vi "题目七.vi"() -> ()   [LabVIEW 2017]
uses:
  <vilib>/Utility/file.llb/Read Delimited Spreadsheet (DBL).vi
  <vilib>/Analysis/NI_AALBase.lvlib
panel:
  out "波形图表":dbl(graph)
  out "all rows":dbl[][](array[numeric]) caption="所有行"
  in  "cycles":dbl=1.0 caption="周期" format="%0.2f"
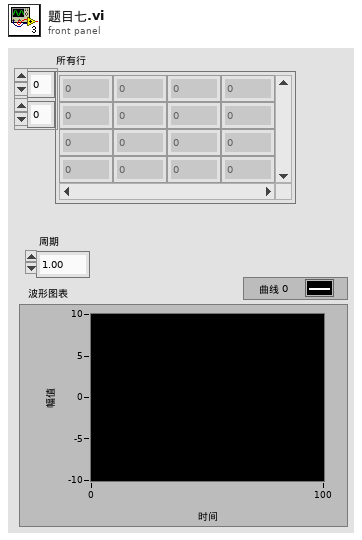
[diagram p1: front panel]
types:
  T1 = enum16{"open", "replace", "create", "open or create", "replace or create", "replace or create with confirmation"}
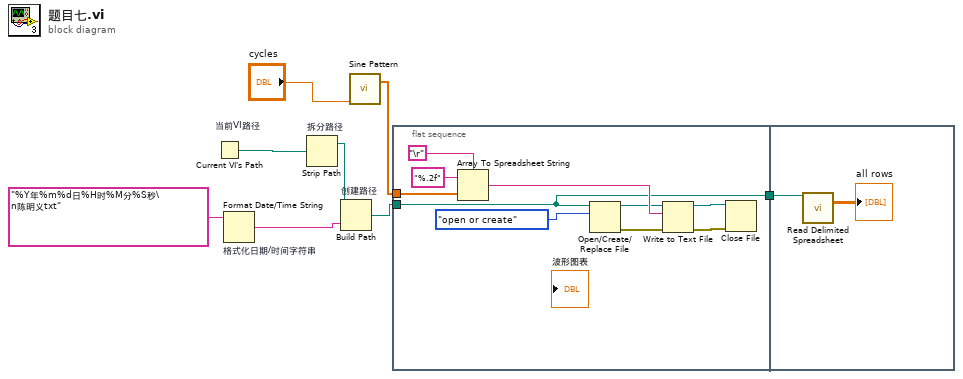
[diagram p0: block diagram]
diagram:
  n1 = Current VI's Path "当前VI路径"() -> (path=w8:path)
  n2 = Format Date/Time String "格式化日期/时间字符串"(time format string (%c)="%Y年%m%d日%H时%M分%S秒\n陈明义txt") -> (date/time string=w7:string)  [unwired: 2 in]
  n3 = Strip Path "拆分路径"(path=w8) -> (stripped path=w6:path)  [unwired: 1 out]
  n4 = Build Path "创建路径"(base path=w6, name or relative path=w7) -> (appended path=w3:path)
  n5 = call <vilib>:"Sine Pattern.vi"("cycles"="cycles") -> ("Sinusoidal Pattern"=w2:dbl[])  [unwired: 3 in, 1 out]
  n6 = flat-sequence {
    tunnel: w3 -> [w10]
    tunnel: w2 -> [w14]
    tunnel: [w10] -> w1
    tunnel: w1 -> [w20]
    frame #0 {
      n7 = Array To Spreadsheet String(delimiter (Tab)="\r", array=w14, 3:"%.2f" ("格式字符串")) -> (spreadsheet string=w11:string)
      n8 = Open/Create/Replace File(file path (use dialog)=w10, operation (0:open)=T1."open or create" ("操作(0:open)")) -> (refnum out=w9:refnum<file>, error out=w18:errorcluster)  [unwired: 4 in, 1 out]
      n9 = Write to Text File(file (use dialog)=w9, text=w11, error in=w18) -> (refnum out=w16:refnum<file>, error out=w17:errorcluster)  [unwired: 1 in, 1 out]
      n10 = Close File(refnum=w16, error in=w17) -> ()  [unwired: 2 out]
    }
    frame #1 {
      n11 = call-poly <vilib>:"Read Delimited Spreadsheet.vi"("file path (dialog if empty)"=w20) -> ("all rows"=→"all rows":dbl[][])  [unwired: 9 in, 5 out]
    }
  }
